vi "Calculate Window Gain.vi"(7 "Onset Indicies":i32[](array[numeric]), 8 "error in (no error)":errorcluster, 9 "Response in":dbl[][](array[numeric]), 10 "Stimulus in":dbl[][](array[numeric]), 11 "Head Impulse Fit in":refnum<class "Head Impulse Fit.lvclass">) -> (0 "error out":errorcluster, 1 "Response out":dbl[][](array[numeric]), 2 "Stimulus out":dbl[][](array[numeric]), 3 "Head Impulse Fit out":refnum<class "Head Impulse Fit.lvclass">)   [LabVIEW 2014, in "Head Impulse Fit.lvclass"]
uses:
  Head Impulse Fit.lvclass
  Head Impulse Fit.lvclass/Head Impulse Fit.ctl
  comm/stats/stats.lvlib
  <vilib>/Analysis/NI_AALBase.lvlib
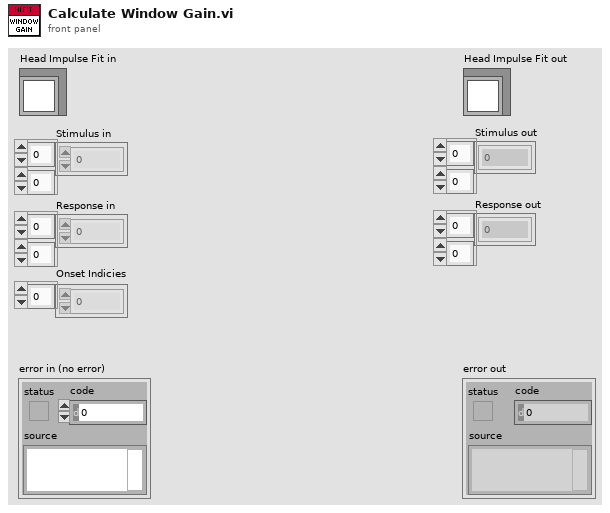
[diagram p1: front panel]
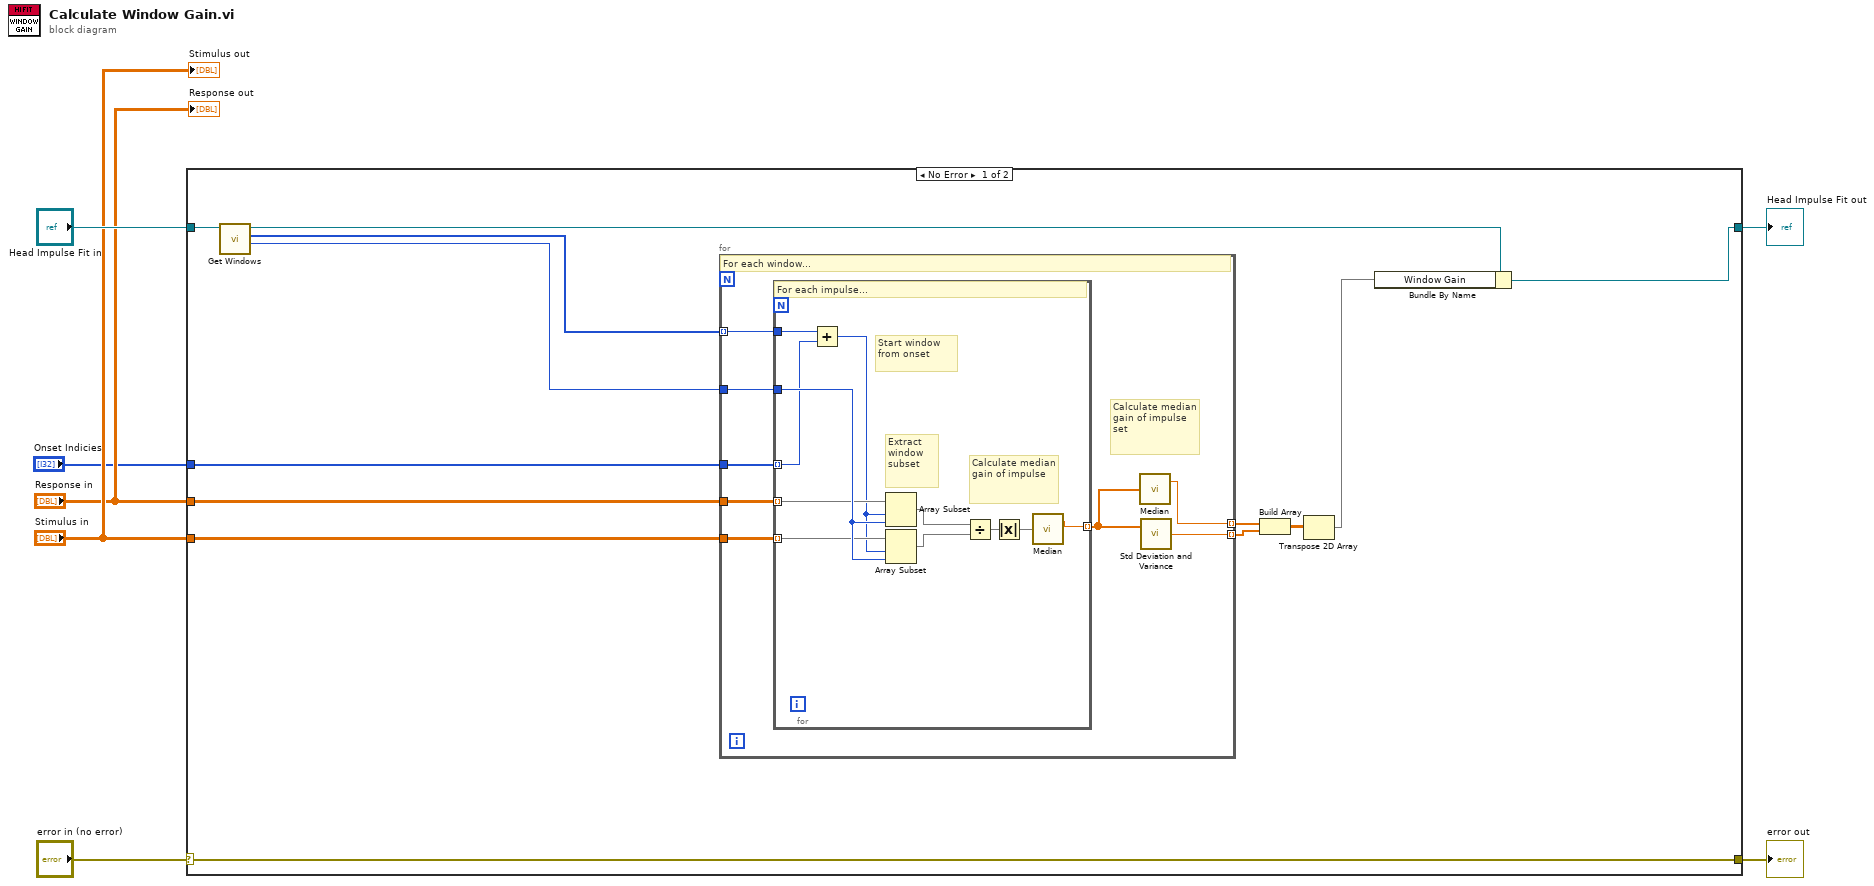
[diagram p0: block diagram]
diagram:
  n1 = case shown="No Error" "error in (no error)" {
    selector: "error in (no error)" -> [w20 w41]
    tunnel: [w20 w41] -> w6
    tunnel: [w13 w40] -> w4
    tunnel: "Head Impulse Fit in" -> [w11 w40]
    tunnel: "Stimulus in" -> [w19 _]
    tunnel: "Response in" -> [w18 _]
    tunnel: "Onset Indicies" -> [w17 _]
    frame No Error {
      n2 = call "Get Windows.vi"("Head Impulse Fit in"=w11) -> ("Window Length"=w8:i32, "Window Start Indicies"=w9:i32[], "Head Impulse Fit out"=w10:refnum<class "Head Impulse Fit.lvclass">)  [unwired: 7 in, 1 out]
      n3 = for {
        tunnel: w8 -> [w28]
        tunnel: w9 -> [w27] mode=indexing
        tunnel: w19 -> [w26]
        tunnel: w18 -> [w25]
        tunnel: w17 -> [w24]
        tunnel: [w21] -> w16 mode=indexing
        tunnel: [w23] -> w15 mode=indexing
        # "Calculate median gain of impulse set"
        # "For each window..."
        n4 = for {
          tunnel: w28 -> [w38]
          tunnel: w27 -> [w39]
          tunnel: w26 -> [w33] mode=indexing
          tunnel: w25 -> [w34] mode=indexing
          tunnel: w24 -> [w31] mode=indexing
          tunnel: [w29] -> w22 mode=indexing
          # "Calculate median gain of impulse"
          # "Extract window\nsubset"
          # "Start window from onset"
          # "For each impulse..."
          n5 = Add(x=w39, y=w31) -> (x+y=w32:i32)
          n6 = Array Subset(array=w34, index=w32, length=w38) -> (w36:dbl[])
          n7 = Array Subset(array=w33, index=w32, length=w38) -> (w35:dbl[])
          n8 = Divide(x=w36, y=w35) -> (x/y=w37:dbl[])
          n9 = Absolute Value(x=w37) -> (abs(x)=w30:dbl[])
          n10 = call <vilib>:"Median.vi"("X"=w30) -> ("median"=w29:dbl)  [unwired: 1 out]
        }
        n11 = call <vilib>:"Median.vi"("X"=w22) -> ("median"=w21:dbl)  [unwired: 1 out]
        n12 = call "Std Deviation and Variance.vi"("X"=w22) -> ("standard deviation"=w23:dbl)  [unwired: 1 in, 2 out]
      }
      n13 = Build Array(w16, w15) -> (w14:dbl[][])
      n14 = Transpose 2D Array(2D array=w14) -> (transposed array=w12:dbl[][])
      n15 = Bundle By Name(cluster=w10, "Window Gain"=w12) -> (w13:refnum<class "Head Impulse Fit.lvclass">)
    }
    frame Error {
    }
  }
  "error out" <- w6
  "Head Impulse Fit out" <- w4
  "Stimulus out" <- "Stimulus in"
  "Response out" <- "Response in"
